vi "Write Single SP.vi"(8 "error in":errorcluster, 10 "sp":sgl caption="Setpoint", 11 "AlicatCommBank in":refnum<class "AlicatCommBank.lvclass">=refnum) -> (0 "error out":errorcluster, 3 "AlicatCommBank out":refnum<class "AlicatCommBank.lvclass">)   [LabVIEW 2014, in "Alicat.lvlib" / "AlicatCommBank.lvclass"]
uses:
  AlicatCommBank.lvclass
  Alicat Controller/Alicat Controller.lvclass
  Alicat.lvclass
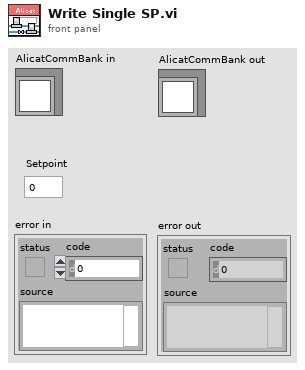
[diagram p1: front panel]
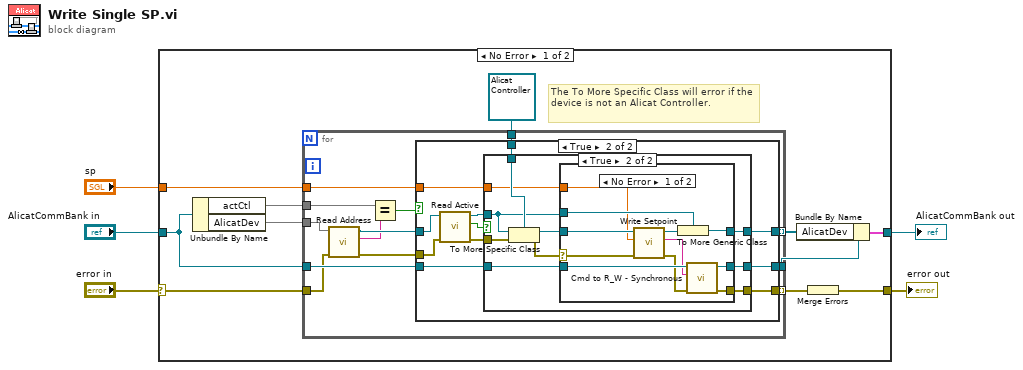
[diagram p0: block diagram]
diagram:
  n1 = case shown="No Error" "error in" {
    selector: "error in" -> [w11 w71]
    tunnel: [w10 w71] -> w5
    tunnel: [w9 w70] -> w4
    tunnel: "AlicatCommBank in" -> [w8 w70]
    tunnel: "sp" -> [w6 _]
    frame No Error {
      # "The To More Specific Class will error if the device is not an Alicat Controller."
      n2 = Unbundle By Name(w8) -> ("actCtl"=w7, "AlicatDev"=w16)
      n3 = for {
        tunnel: w8 -> [w25]
        tunnel: [w29] -> w14
        tunnel: [w28] -> w12 mode=indexing
        tunnel: w11 -> [w24]
        tunnel: w16 -> [w22]
        tunnel: refnum<class "Alicat Controller.lvclass"> refnum ("Alicat Controller.lvclass") -> [w27]
        tunnel: [w26] -> w13 mode=indexing
        tunnel: w7 -> [w19]
        tunnel: w6 -> [w17]
        n4 = call "Read Address.vi"("error in"=w24, "Alicat in"=w22) -> ("error out"=w23:errorcluster, "Address"=w20:string, "Alicat out"=w21:refnum<class "Alicat.lvclass">)  [unwired: 7 in]
        n5 = Equal?(x=w19, y=w20) -> (x = y?=w18:bool)
        n6 = case shown="True" w18 {
          tunnel: [w31 w43] -> w29
          tunnel: [w30 w42] -> w28
          tunnel: w27 -> [_ w41]
          tunnel: [w32 w40] -> w26
          tunnel: w25 -> [w31 w39]
          tunnel: w23 -> [w30 w35]
          tunnel: w21 -> [w32 w37]
          tunnel: w17 -> [_ w38]
          frame False {
          }
          frame True {
            n7 = call "Read Active.vi"("error in"=w35, "Alicat in"=w37) -> ("error out"=w34:errorcluster, "Active?"=w33:bool, "Alicat out"=w36:refnum<class "Alicat.lvclass">)  [unwired: 7 in]
            n8 = case shown="True" w33 {
              tunnel: [w45 w56] -> w43
              tunnel: [w44 w55] -> w42
              tunnel: w41 -> [_ w54]
              tunnel: [w46 w51] -> w40
              tunnel: w39 -> [w45 w50]
              tunnel: w38 -> [_ w49]
              tunnel: w36 -> [w46 w48]
              tunnel: w34 -> [w44 w47]
              frame False {
              }
              frame True {
                n9 = To More Specific Class(target class=w54, reference=w48, error in=w47) -> (specific class reference=w53:refnum<class "Alicat Controller.lvclass">, error out=w52:errorcluster)
                n10 = case shown="No Error" w52 {
                  selector: w52 -> [w63 _]
                  tunnel: w50 -> [w67 w69]
                  tunnel: [w66 w69] -> w56
                  tunnel: [w65 _] -> w55
                  tunnel: w53 -> [w64 _]
                  tunnel: [w62 w68] -> w51
                  tunnel: w48 -> [w61 w68]
                  tunnel: w49 -> [w57 _]
                  frame No Error {
                    n11 = call "Write Setpoint.vi"("error in"=w63, "Setpoint"=w57, "Alicat Controller in"=w64) -> ("error out"=w59:errorcluster, "SPStr"=w60:string, "Alicat Controller out"=w58:refnum<class "Alicat Controller.lvclass">)  [unwired: 6 in]
                    n12 = To More Generic Class(target class=w61, reference=w58) -> (generic class reference=w62:refnum<class "Alicat.lvclass">)
                    n13 = call-dynamic "Cmd to R_W - Synchronous.vi"("error in"=w59, "write buffer"=w60, "Serial IO in"=w67) -> ("error out"=w65:errorcluster, "Serial IO out"=w66:refnum<class "AlicatCommBank.lvclass">)  [unwired: 6 in, 1 out]
                  }
                  frame Error {
                    # "Not a controller"
                  }
                }
              }
            }
          }
        }
      }
      n14 = Bundle By Name(cluster=w14, "AlicatDev"=w13) -> (w9:cluster{})
      n15 = Merge Errors(w12) -> (w10:errorcluster)
    }
    frame Error {
    }
  }
  "error out" <- w5
  "AlicatCommBank out" <- w4
